vi "Read - Read Me File.vi"() -> (2 "full text":string, 3 "Version":string)   [LabVIEW 2018]
panel:
  out "error out":errorcluster
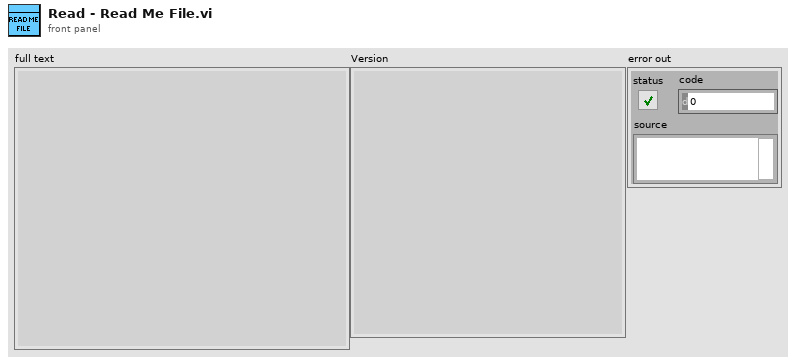
[diagram p1: front panel]
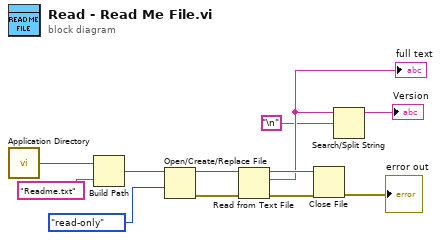
[diagram p0: block diagram]
diagram:
  n1 = call <vilib>:"Application Directory.vi"() -> ("Application Directory"=w12:path)
  n2 = Build Path(base path=w12, name or relative path="Readme.txt") -> (appended path=w10:path)
  n3 = Open/Create/Replace File(file path (use dialog)=w10, access (0:read/write)=enum16{"read/write", "read-only", "write-only"}."read-only") -> (refnum out=w9:refnum<file>, error out=w8:errorcluster)  [unwired: 4 in, 1 out]
  n4 = Read from Text File(file (use dialog)=w9, error in=w8) -> (refnum out=w6:refnum<file>, text=w5:string, error out=w7:errorcluster)  [unwired: 2 in, 1 out]
  "full text" <- w5
  n5 = Close File(refnum=w6, error in=w7) -> (error out=→"error out":errorcluster)  [unwired: 1 out]
  n6 = Search/Split String(string=w5, search string/char (-)="\n") -> (substring before match=→"Version":string)  [unwired: 1 in, 2 out]
